vi "Shift Cartesian Axes.vi"(1 "Coordinate Offset":dbl[](array[numeric]), 2 "Coordinate Switch":bool, 3 "Coordinate Input":dbl[](array[numeric]), 4 "Direction":enum16{" +", " - "}(ring)) -> (0 "Coordinate Output":dbl[](array[numeric]))   [LabVIEW 2009]
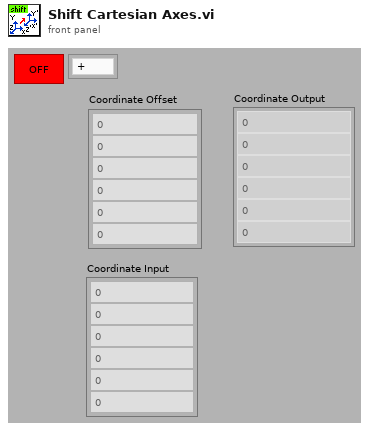
[diagram p1: front panel]
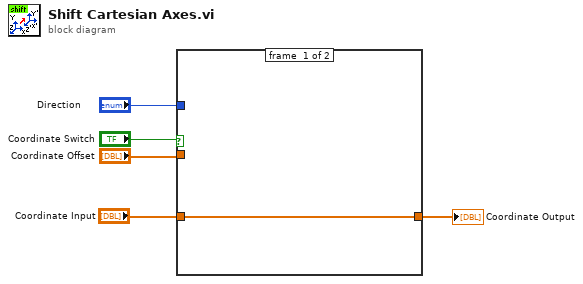
[diagram p0: block diagram]
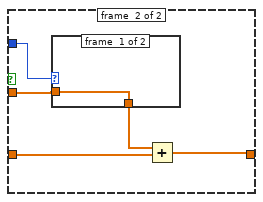
[diagram p2: hidden frame]
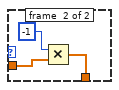
[diagram p3: hidden frame]
diagram:
  n1 = case shown="True" "Coordinate Switch" {
    tunnel: "Coordinate Offset" -> [_ w8]
    tunnel: "Direction" -> [_ w7]
    tunnel: [w6 w11] -> w1
    tunnel: "Coordinate Input" -> [w6 w10]
    frame #0 {
    }
    frame #1 {
      n2 = case shown="\" +\"" w7 {
        tunnel: w8 -> [w12 w15]
        tunnel: [w12 w13] -> w9
        frame #0 {
        }
        frame #1 {
          n3 = Multiply(x=-1, y=w15) -> (x*y=w13:dbl[])
        }
      }
      n4 = Add(x=w9, y=w10) -> (x+y=w11:dbl[])
    }
  }
  "Coordinate Output" <- w1
